vi "Lab Panel V5.26.vi"() -> ()   [LabVIEW 2017]
uses:
  <vilib>/platform/TimedLoop/XDataNode/XDataNode.xnode
  <vilib>/Platform/TimedLoop/XDataNode/nitl_modes.ctl
  <vilib>/Platform/TimedLoop/XDataNode/XDNodeRunTimeDep.lvlib
  <vilib>/Platform/TimedLoop/XDataNode/wakeup.ctl
  <vilib>/Platform/TimedLoop/XDataNode/timing_clust.ctl
  Global 1.vi
  Global display 1.vi
  Global display 3.vi
  Global display 2.vi
  Global display 4.vi
panel:
  out "Simulate IND":bool
  out "Amb Tp":dbl format="%#.0f"
  out "Tp Up":dbl
  out "network error":bool
  out "TEMP":bool
  out "AI":bool
  in  "stop all":bool
  in  "ADMIN":bool
  in  "Tab Control 2":T1(tab)
  out "SIG LAB05-2":T2 {"PF" format="%.2f"; "AMPS" format="%.1f"}
  out "SIG LAB05-1":T2 {"PF" format="%.2f"; "AMPS" format="%.1f"}
  out "SIG LAB04-2":T2 {"PF" format="%.2f"; "AMPS" format="%.1f"}
  out "SIG LAB04-1":T2 {"PF" format="%.2f"; "AMPS" format="%.1f"}
  out "SIG LAB03-2":T2 {"PF" format="%.2f"; "AMPS" format="%.1f"}
  out "SIG LAB03-1":T2 {"PF" format="%.2f"; "AMPS" format="%.1f"}
  out "SIG LAB02-2":T2 {"PF" format="%.2f"; "AMPS" format="%.1f"}
  in  "RUN LAB01-1":bool
  in  "O/I  LAB05-1":bool
  in  "O/I  LAB05-2":bool
  in  "O/I  LAB04-1":bool
  in  "O/I  LAB04-2":bool
  in  "O/I  LAB02-1":bool
  in  "O/I  LAB02-2":bool
  in  "O/I  LAB01-2":bool
  in  "O/I  LAB01-1":bool
  in  "O/I  LAB03-1":bool
  in  "RUN LAB05-2":bool
  in  "RUN LAB05-1":bool
  in  "RUN LAB04-2":bool
  in  "RUN LAB04-1":bool
  in  "RUN LAB03-2":bool
  in  "RUN LAB03-1":bool
  in  "RUN LAB02-2":bool
  in  "RUN LAB02-1":bool
  in  "RUN LAB01-2":bool
  in  "SELECT LAB05-2":T3(radio)
  in  "SELECT LAB05-1":T3(radio)
  in  "SELECT LAB04-2":T3(radio)
  in  "SELECT LAB04-1":T3(radio)
  in  "SELECT LAB03-2":T3(radio)
  in  "SELECT LAB03-1":T3(radio)
  in  "SELECT LAB02-2":T3(radio)
  in  "SELECT LAB02-1":T3(radio)
  in  "SELECT LAB01-2":T3(radio)
  in  "SELECT LAB01-1":T3(radio)
  in  "O/I  LAB03-2":bool
  out "SIG LAB01-1":T2 {"PF" format="%.2f"; "AMPS" format="%.1f"}
  out "SIG LAB01-2":T2 {"PF" format="%.2f"; "AMPS" format="%.1f"}
  out "SIG LAB02-1":T2 {"PF" format="%.2f"; "AMPS" format="%.1f"}
  out "DISP LAB05-2":T4 {"MINS" format="%.2g"}
  out "DISP LAB05-1":T4 {"MINS" format="%.2g"}
  out "DISP LAB04-2":T4 {"MINS" format="%.2g"}
  out "DISP LAB04-1":T4 {"MINS" format="%.2g"}
  out "DISP LAB03-2":T4 {"MINS" format="%.2g"}
  out "DISP LAB03-1":T4 {"MINS" format="%.2g"}
  in  "SET LAB05-2":T5={"NAME"="", "DESCRIPTION"="", "CYCLES"=5.0, "T-RISE mins"=0.0, "T-RISE deg C"=0.0} {"CYCLES" min=5.0 step=1.0}
  in  "SET LAB05-1":T5={"NAME"="", "DESCRIPTION"="", "CYCLES"=5.0, "T-RISE mins"=0.0, "T-RISE deg C"=0.0} {"CYCLES" min=5.0 step=1.0}
  in  "SET LAB04-2":T5={"NAME"="", "DESCRIPTION"="", "CYCLES"=5.0, "T-RISE mins"=0.0, "T-RISE deg C"=0.0} {"CYCLES" min=5.0 step=1.0}
  in  "SET LAB04-1":T5={"NAME"="", "DESCRIPTION"="", "CYCLES"=5.0, "T-RISE mins"=0.0, "T-RISE deg C"=0.0} {"CYCLES" min=5.0 step=1.0}
  in  "SET LAB03-2":T5={"NAME"="", "DESCRIPTION"="", "CYCLES"=5.0, "T-RISE mins"=0.0, "T-RISE deg C"=0.0} {"CYCLES" min=5.0 step=1.0}
  in  "SET LAB03-1":T5={"NAME"="", "DESCRIPTION"="", "CYCLES"=5.0, "T-RISE mins"=0.0, "T-RISE deg C"=0.0} {"CYCLES" min=5.0 step=1.0}
  out "DISP LAB02-2":T4 {"MINS" format="%.2g"}
  out "DISP LAB02-1":T4 {"MINS" format="%.2g"}
  in  "SET LAB02-2":T5={"NAME"="", "DESCRIPTION"="", "CYCLES"=5.0, "T-RISE mins"=0.0, "T-RISE deg C"=0.0} {"CYCLES" min=5.0 step=1.0}
  in  "SET LAB02-1":T5={"NAME"="", "DESCRIPTION"="", "CYCLES"=5.0, "T-RISE mins"=0.0, "T-RISE deg C"=0.0} {"CYCLES" min=5.0 step=1.0}
  out "RESULT LAB05-2":bool
  out "RESULT LAB05-1":bool
  out "RESULT LAB04-2":bool
  out "RESULT LAB04-1":bool
  out "RESULT LAB03-2":bool
  out "RESULT LAB03-1":bool
  out "RESULT LAB02-2":bool
  out "RESULT LAB02-1":bool
  out "RESULT LAB01-2":bool
  out "RESULT LAB01-1":bool
  in  "SET LAB01-1":T5={"NAME"="", "DESCRIPTION"="", "CYCLES"=5.0, "T-RISE mins"=0.0, "T-RISE deg C"=0.0} {"CYCLES" min=5.0 step=1.0}
  in  "SET LAB01-2":T5={"NAME"="", "DESCRIPTION"="", "CYCLES"=5.0, "T-RISE mins"=0.0, "T-RISE deg C"=0.0} {"CYCLES" min=5.0 step=1.0}
  out "DISP LAB01-1":T4 {"MINS" format="%.2g"}
  out "DISP LAB01-2":T4 {"MINS" format="%.2f"}
  out "TEMP RISE LAB05-2":cluster{"TL":dbl, "TN":dbl}
  out "TEMP RISE LAB05-1":cluster{"TL":dbl, "TN":dbl}
  out "TEMP RISE LAB04-2":cluster{"TL":dbl, "TN":dbl}
  out "TEMP RISE LAB04-1":cluster{"TL":dbl, "TN":dbl}
  out "TEMP RISE LAB03-2":cluster{"TL":dbl, "TN":dbl}
  out "TEMP RISE LAB03-1":cluster{"TL":dbl, "TN":dbl}
  out "TEMP RISE LAB02-2":cluster{"TL":dbl, "TN":dbl}
  out "TEMP RISE LAB02-1":cluster{"TL":dbl, "TN":dbl}
  out "TEMP RISE LAB01-2":cluster{"TL":dbl, "TN":dbl}
  out "TEMP RISE LAB01-1":cluster{"TL":dbl, "TN":dbl}
  out "JIG LAB05-2":bool
  out "JIG LAB05-1":bool
  out "JIG LAB04-2":bool
  out "JIG LAB04-1":bool
  out "JIG LAB03-2":bool
  out "JIG LAB03-1":bool
  out "JIG LAB02-2":bool
  out "JIG LAB02-1":bool
  out "JIG LAB01-2":bool
  out "JIG LAB01-1":bool
  out "TEMP START LAB01-1":cluster{"TL":dbl, "TN":dbl}
  out "TEMP START LAB02-1":cluster{"TL":dbl, "TN":dbl}
  out "TEMP START LAB03-1":cluster{"TL":dbl, "TN":dbl}
  out "TEMP START LAB04-1":cluster{"TL":dbl, "TN":dbl}
  out "TEMP START LAB01-2":cluster{"TL":dbl, "TN":dbl}
  out "TEMP START LAB02-2":cluster{"TL":dbl, "TN":dbl}
  out "TEMP START LAB03-2":cluster{"TL":dbl, "TN":dbl}
  out "TEMP START LAB04-2":cluster{"TL":dbl, "TN":dbl}
  out "TEMP START LAB05-2":cluster{"TL":dbl, "TN":dbl}
  out "TEMP START LAB05-1":cluster{"TL":dbl, "TN":dbl}
  out "LOG LAB05-2":string
  out "LOG LAB04-2":string
  out "LOG LAB03-2":string
  out "LOG LAB02-2":string
  out "LOG LAB01-2":string
  out "LOG LAB05-1":string
  out "LOG LAB04-1":string
  out "LOG LAB03-1":string
  out "LOG LAB02-1":string
  out "LOG LAB01-1":string
  in  "Tab charts":T6(tab)
  out "LAB01 VOLTS":dynamicdata(graph)
  out "LAB01 AMPS":dynamicdata(graph)
  out "LAB01 deg C":dynamicdata(graph)
  out "LAB02 VOLTS":dynamicdata(graph)
  out "LAB02 AMPS":dynamicdata(graph)
  out "LAB02 deg C":dynamicdata(graph)
  out "LAB03 VOLTS":dynamicdata(graph)
  out "LAB03 AMPS":dynamicdata(graph)
  out "LAB03 deg C":dynamicdata(graph)
  out "LAB04 VOLTS":dynamicdata(graph)
  out "LAB04 AMPS":dynamicdata(graph)
  out "LAB04 deg C":dynamicdata(graph)
  out "LAB05 VOLTS":dynamicdata(graph)
  out "LAB05 AMPS":dynamicdata(graph)
  out "LAB05 deg C":dynamicdata(graph)
  out "Reset Error":bool
  out "Error Temp":bool
  out "Er USB#2":dbl
  out "Er USB#1":dbl
  out "Er USB#0":dbl
  out "Resets Done":dbl
  out "Error USB #2":bool
  out "Error USB #1":bool
  out "Error USB #0":bool
  in  "MAIL SETTINGS":T7
  out "MAIL REPORT":string
  in  "TO (string):":string
  in  "Send Mail Now":bool
  in  "Auto Mail Send":bool
  in  "Network Directory":path
  in  "JIG ON TIME (S)":dbl=1.0 min=1.0 max=10.0 step=0.5 format="%.1g"
  in  "JIG OFF TIME (S)":dbl=2.0 min=2.0 max=10.0 step=0.5 format="%.1g"
  in  "Reset Measuring":bool
  in  "Read Temp":bool
  out "JIG RELAY CYCLES":T8
  out "ON L05-2":cluster{"amps":dbl, "volts":dbl, "pf":dbl}
  out "ON L05-1":cluster{"amps":dbl, "volts":dbl, "pf":dbl}
  out "FAIL LAB05-2":cluster{"LO":dbl, "HI":dbl}
  out "FAIL LAB05-1":cluster{"LO":dbl, "HI":dbl}
  out "FAIL LAB04-2":cluster{"LO":dbl, "HI":dbl}
  out "FAIL LAB04-1":cluster{"LO":dbl, "HI":dbl}
  out "FAIL LAB03-2":cluster{"LO":dbl, "HI":dbl}
  out "FAIL LAB03-1":cluster{"LO":dbl, "HI":dbl}
  out "FAIL LAB02-2":cluster{"LO":dbl, "HI":dbl}
  out "FAIL LAB02-1":cluster{"LO":dbl, "HI":dbl}
  out "FAIL LAB01-2":cluster{"LO":dbl, "HI":dbl}
  out "FAIL LAB01-1":cluster{"LO":dbl, "HI":dbl}
  out "ON L01-1":cluster{"amps":dbl, "volts":dbl, "pf":dbl}
  out "ON L01-2":cluster{"amps":dbl, "volts":dbl, "pf":dbl}
  out "ON L02-1":cluster{"amps":dbl, "volts":dbl, "pf":dbl}
  out "ON L02-2":cluster{"amps":dbl, "volts":dbl, "pf":dbl}
  out "ON L03-1":cluster{"amps":dbl, "volts":dbl, "pf":dbl}
  out "ON L03-2":cluster{"amps":dbl, "volts":dbl, "pf":dbl}
  out "ON L04-1":cluster{"amps":dbl, "volts":dbl, "pf":dbl}
  out "ON L04-2":cluster{"amps":dbl, "volts":dbl, "pf":dbl}
  out "TEMP LA05":T9
  out "TEMP LA04":T9
  out "TEMP LA03":T9
  out "TEMP LA02":T9
  out "TEMP LA01":T9
  out "Ref deg C":dbl format="%#.0f"
  out "Temp read loop":dbl
  out "AI Task":bool
  out "AI Task2":dbl
  out "AI Task1":dbl
  out "AI Task0":dbl
  out "Total USB resets":dbl
  in  "Auto Reset":bool
  in  "Mail Test File To:":string
  in  "Mail Test Fail":bool
  out "graph flag":bool
  in  "Temp Test Cal":dbl
  in  "Amps Fail level":dbl
  in  "Fail Loops":dbl
  out "Save JC":bool
  in  "Simulate":bool
  in  "Temp Value":dbl
  in  "Temp Delay Lps":dbl
  in  "SAMPLES":dbl
  in  "RATE (Hz)":dbl
  in  "JIG TEST":T10
  in  "C drive data root dir":path
  out "run lab05-2":bool
  out "run lab05-1":bool
  out "run lab04-2":bool
  out "run lab04-1":bool
  out "run lab03-2":bool
  out "run lab03-1":bool
  out "run lab02-2":bool
  out "run lab02-1":bool
  out "run lab01-2":bool
  out "run lab01-1":bool
  in  "Tab Control":T11(tab)
  out "LAB01-2 (GRAPH)":dynamicdata(graph)
  out "LAB01-1 (GRAPH)":dynamicdata(graph)
  out "LAB02-2 (GRAPH)":dynamicdata(graph)
  out "LAB02-1 (GRAPH)":dynamicdata(graph)
  out "LAB03-2 (GRAPH)":dynamicdata(graph)
  out "LAB03-1 (GRAPH)":dynamicdata(graph)
  out "LAB04-2 (GRAPH)":dynamicdata(graph)
  out "LAB04-1 (GRAPH)":dynamicdata(graph)
  out "LAB05-2 (GRAPH)":dynamicdata(graph)
  out "LAB05-1 (GRAPH)":dynamicdata(graph)
  out "Any Test Running":bool
  out "Read Time":dbl
  out "LAB05 TEMP":T12
  out "LAB04 TEMP":T12
  out "LAB02 TEMP":T12
  out "LAB01 TEMP":T12
  out "LAB03 TEMP":T12
  out "LAB05-TP":bool
  out "LAB04-TP":bool
  out "LAB03-TP":bool
  out "LAB02-TP":bool
  out "LAB01-TP":bool
  out "Analog error":bool
  out "USB OUT 0":bool[](array[boolean])
  out "USB OUT 1":bool[](array[boolean])
  out "USB OUT 2":bool[](array[boolean])
  in  "Ambient Volts":dbl format="%.2f"
  in  "PF":dbl min=0.0 max=1.0 step=0.1 format="%#.1f"
  in  "VOLTS":dbl
  in  "OFF amps":dbl min=0.0 max=100.0 step=0.1 format="%#.1f"
  in  "ON amps":dbl
  in  "LAB deg C":T13
  out "AI data 0":waveform(dbl)[](array[waveform])
  out "AI data 1":waveform(dbl)[](array[waveform])
  out "AI data 2":waveform(dbl)[](array[waveform])
  out "AI Error":errorcluster[](array[cluster])
  out "AI loop time":dbl format="%.6g"
  out "loops":dbl
  in  "SAMPLES 2":dbl
  out "on loops":dbl format="%#.0f"
  out "off loops":dbl format="%#.0f"
  out "jig cycle":dbl
  out "TDMS LAB01-1":refnum<k34>
  out "data file error":errorcluster
  out "TDMS LAB02-1":refnum<k34>
  out "TDMS LAB01-2":refnum<k34>
  out "TDMS LAB02-2":refnum<k34>
  out "TDMS LAB03-1":refnum<k34>
  out "TDMS LAB03-2":refnum<k34>
  out "TDMS LAB04-1":refnum<k34>
  out "TDMS LAB04-2":refnum<k34>
  out "TDMS LAB05-1":refnum<k34>
  out "TDMS LAB05-2":refnum<k34>
  out "mail control":string
  out "File Time Stamp":timestamp
  in  "stop":bool
  in  "Select COM port":refnum<visa-resource-name>="COM6"
  out "COM port":refnum<visa-resource-name>="COM6"
  out "deg C (volts)":dbl
  out "TEMP REF cal":dbl
  out "CAL LAB01":T14 {"2 (TN) cal" min=0.0 step=0.01 format="%.2f"; "2 (TL) cal" min=0.0 step=0.01 format="%.2f"; "2 (PF) cal" min=0.0 step=0.01 format="%.2f"; "2 (V) cal" min=0.0 step=0.01 format="%.2f"; "2 (A) cal" min=0.0 step=0.01 format="%.2f"; "1 (TN) cal" min=0.0 step=0.01 format="%.2f"; "1 (TL) cal" min=0.0 step=0.01 format="%.2f"; "1 (PF) cal" min=0.0 step=0.01 format="%.2f"; "1 (V) cal" min=0.0 step=0.01 format="%.2f"; "1  (A) cal" min=0.0 step=0.01 format="%.2f"}
  out "CAL LAB03":T14 {"2 (TN) cal" min=0.0 step=0.01 format="%.2f"; "2 (TL) cal" min=0.0 step=0.01 format="%.2f"; "2 (PF) cal" min=0.0 step=0.01 format="%.2f"; "2 (V) cal" min=0.0 step=0.01 format="%.2f"; "2 (A) cal" min=0.0 step=0.01 format="%.2f"; "1 (TN) cal" min=0.0 step=0.01 format="%.2f"; "1 (TL) cal" min=0.0 step=0.01 format="%.2f"; "1 (PF) cal" min=0.0 step=0.01 format="%.2f"; "1 (V) cal" min=0.0 step=0.01 format="%.2f"; "1  (A) cal" min=0.0 step=0.01 format="%.2f"}
  out "CAL LAB02":T15 {"2 (TN) cal" min=0.0 step=0.01 format="%.2f"; "2 (TL) cal" min=0.0 step=0.01 format="%.2f"; "2 (PF) cal" min=0.0 step=0.01 format="%.2f"; "2 (V) cal" min=0.0 step=0.01 format="%.2f"; "2 (A) cal" min=0.0 step=0.01 format="%.2f"; "1 (TN) cal" min=0.0 step=0.01 format="%.2f"; "1 (TL) cal" min=0.0 step=0.01 format="%.2f"; "1 (PF) cal" min=0.0 step=0.01 format="%.2f"; "1 (V) cal" min=0.0 step=0.01 format="%.2f"; "1 (A) cal" min=0.0 step=0.01 format="%.2f"}
  out "CAL LAB05":T14 {"2 (TN) cal" min=0.0 step=0.01 format="%.2f"; "2 (TL) cal" min=0.0 step=0.01 format="%.2f"; "2 (PF) cal" min=0.0 step=0.01 format="%.2f"; "2 (V) cal" min=0.0 step=0.01 format="%.2f"; "2 (A) cal" min=0.0 step=0.01 format="%.2f"; "1 (TN) cal" min=0.0 step=0.01 format="%.2f"; "1 (TL) cal" min=0.0 step=0.01 format="%.2f"; "1 (PF) cal" min=0.0 step=0.01 format="%.2f"; "1 (V) cal" min=0.0 step=0.01 format="%.2f"; "1  (A) cal" min=0.0 step=0.01 format="%.2f"}
  out "CAL LAB04":T14 {"2 (TN) cal" min=0.0 step=0.01 format="%.2f"; "2 (TL) cal" min=0.0 step=0.01 format="%.2f"; "2 (PF) cal" min=0.0 step=0.01 format="%.2f"; "2 (V) cal" min=0.0 step=0.01 format="%.2f"; "2 (A) cal" min=0.0 step=0.01 format="%.2f"; "1 (TN) cal" min=0.0 step=0.01 format="%.2f"; "1 (TL) cal" min=0.0 step=0.01 format="%.2f"; "1 (PF) cal" min=0.0 step=0.01 format="%.2f"; "1 (V) cal" min=0.0 step=0.01 format="%.2f"; "1  (A) cal" min=0.0 step=0.01 format="%.2f"}
  out "cal file error out":errorcluster
  in  "SET (cal)":bool
  out "AI Data 0":waveform(dbl)[](graph)
  out "AI Data 1":waveform(dbl)[](graph)
  out "AI Data 2":waveform(dbl)[](graph)
  # "LAB01"
  # "LAB02"
  # "LAB03"
  # "LAB04"
  # "LAB05"
  # "LAB01"
  # "LAB02"
  # "LAB03"
  # "LAB04"
  # "LAB05"
  # "PANEL ID / DATE / TIME / NAME / DESCRIPTION / CYCLES / TEST TIME / STATUS"
  # "PANEL ID / DATE / TIME / NAME / DESCRIPTION / CYCLES / TEST TIME / STATUS"
  # "(Enter recipients address seperated by comma)"
  # "JIG SET"
  # "Temperature circuits \ndetected at start up."
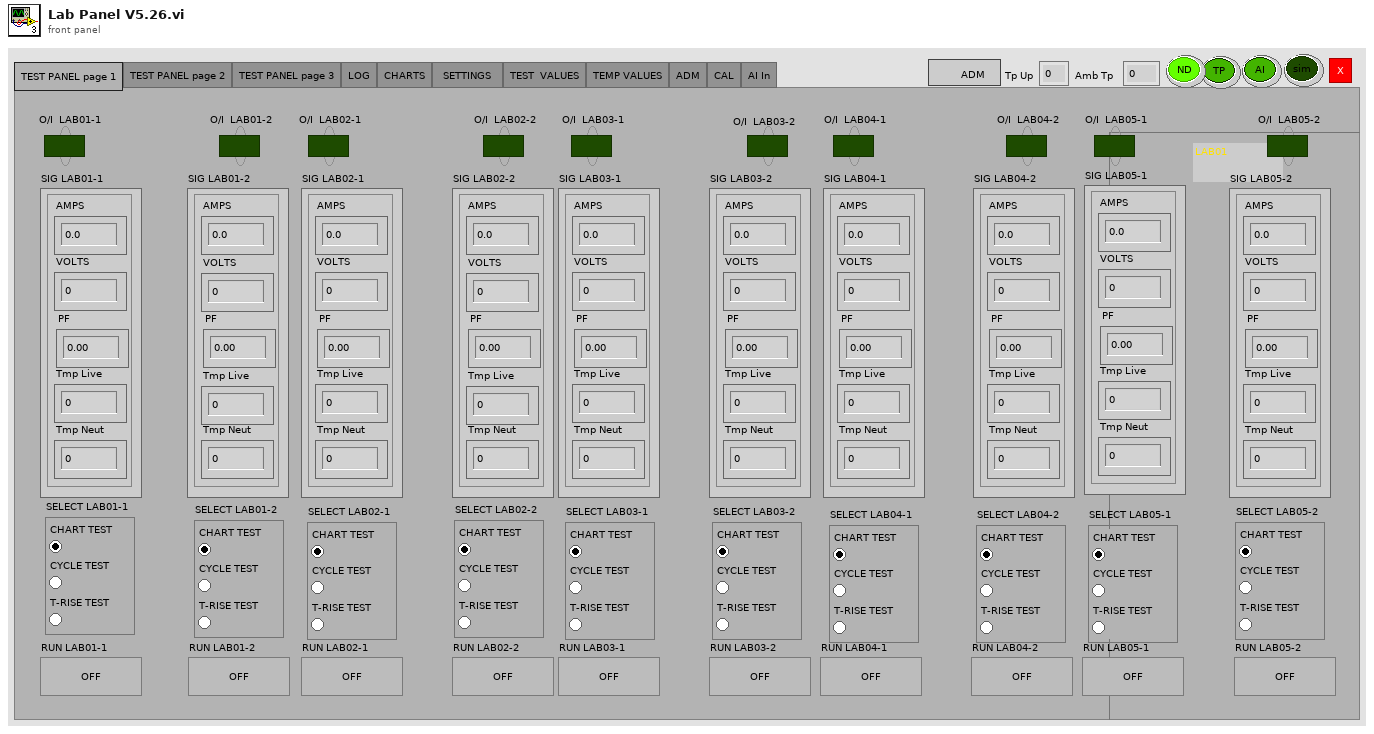
[diagram p1: front panel]
types:
  T1 = enum32{"TEST PANEL page 1", "TEST PANEL page 2", "TEST PANEL page 3", "LOG", "CHARTS", "SETTINGS   ", "TEST  VALUES", "TEMP VALUES", "ADM", "CAL", "AI In"}
  T2 = cluster{"AMPS":dbl, "VOLTS":dbl, "PF":dbl, "Tmp Live":dbl, "Tmp Neut":dbl}
  T3 = enum32{"CHART TEST", "CYCLE TEST", "T-RISE TEST"}
  T4 = cluster{"CYCLE":dbl, "MINS":dbl, "STATUS":string}
  T5 = cluster{"NAME":string, "DESCRIPTION":string, "CYCLES":dbl, "T-RISE mins":dbl, "T-RISE deg C":dbl}
  T6 = enum32{"LAB01", "LAB02", "LAB03", "LAB04", "LAB05"}
  T7 = cluster{"OUT SERVER ADDRESS":string, "FROM ACCOUNT":string, "USER NAME":string, "PASSWORD":string, "TEST MAIL":bool, "TEST MAIL STATUS":string, "mail error":errorcluster}
  T8 = cluster{"LAB01-1":dbl, "LAB01-2":dbl, "LAB02-1":dbl, "LAB02-2":dbl, "LAB03-1":dbl, "LAB03-2":dbl, "LAB04-1":dbl, "LAB04-2":dbl, "LAB05-1":dbl, "LAB05-2":dbl}
  T9 = cluster{"TL-1":dbl, "TN-1":dbl, "TL-2":dbl, "TN-2":dbl, "TL -1COUNT":dbl, "TN-1 COUNT":dbl, "TL-2 COUNT":dbl, "TN-2 COUNT":dbl}
  T10 = cluster{" LAB01-1":bool, " LAB01-2":bool, "LAB02-1":bool, " LAB02-2":bool, "LAB03-1":bool, "LAB03-2":bool, "LAB04-1":bool, "LAB04-2":bool, "LAB05-1":bool, "LAB05-2":bool}
  T11 = enum32{"LAB01", "LAB02", "LAB03", "LAB04", "LAB05", "TEMPERATURE", "GENERAL INFO", "Simulate", "AI Data Out"}
  T12 = cluster{"T1 Live":dbl, "T1 Neut":dbl, "T2 Live":dbl, "T2 Neut":dbl, "ID":dbl, "ER":dbl}
  T13 = cluster{"1 TL":dbl, "1 TN":dbl, "2 TL":dbl, "2 TN":dbl, "ID":dbl, "ER":dbl}
  T14 = cluster{"1  (A) cal":dbl, "1 (V) cal":dbl, "1 (PF) cal":dbl, "1 (TL) cal":dbl, "1 (TN) cal":dbl, "2 (A) cal":dbl, "2 (V) cal":dbl, "2 (PF) cal":dbl, "2 (TL) cal":dbl, "2 (TN) cal":dbl}
  T15 = cluster{"1 (A) cal":dbl, "1 (V) cal":dbl, "1 (PF) cal":dbl, "1 (TL) cal":dbl, "1 (TN) cal":dbl, "2 (A) cal":dbl, "2 (V) cal":dbl, "2 (PF) cal":dbl, "2 (TL) cal":dbl, "2 (TN) cal":dbl}
  T16 = enum8{"Enabled", "Disabled", "Disabled and Grayed Out"}
  T17 = enum16{"open", "replace", "create", "open or create", "replace or create", "replace or create with confirmation"}
  T18 = typedef "XDNodeRunTimeDep.lvlib/timing_clust.ctl" = cluster{"Expected End [f-1]":u64, "Actual End [f-1]":u64, "Finished Late? [f-1]":bool, "Expected End [i-1]":u64, "Actual End [i-1]":u64, "Finished Late? [i-1]":bool, "Expected Start [i]":u64, "Actual Start [i]":u64, "Expected Start [f]":u64, "Actual Start [f]":u64, "Source Name":string, "Structure Name":string, "Period":i64, "Deadline":i64, "Offset":i64, "Start":i64, "Priority":i32, "Timeout":i32, "Mode":T19, "Wakeup Reason":T20, "Error":errorcluster, "Source Type":string, "Secondary Source Type":string, "Global End Time":u64, "Global Start Time":u64, "Frame Duration":u64, "Iteration Duration":u64, "Assigned CPU":i32, "I/O Scan Engine Mode":u32}
  T19 = typedef "XDNodeRunTimeDep.lvlib/nitl_modes.ctl" = enum32{"No Change", "Process missed periods, maintain original phase", "Discard missed periods, maintain original phase", "Process missed periods, ignore original phase", "Discard missed periods, ignore original phase"}
  T20 = typedef "XDNodeRunTimeDep.lvlib/wakeup.ctl" = enum32{"Normal", "Aborted", "Asynchronous wakeup", "Timing source error", "Timed loop error", "Timeout"}
  T21 = enum16{"open", "open or create", "create or replace", "create", "open (read-only)"}
  T22 = cluster{"SET LAB01-1":cluster{"NAME":string, "DESCRIPTION":string, "CYCLES":dbl, "T-RISE mins":dbl, "T-RISE deg C":dbl}, "SET LAB01-2":cluster{"NAME":string, "DESCRIPTION":string, "CYCLES":dbl, "T-RISE mins":dbl, "T-RISE deg C":dbl}, "SET LAB02-1":cluster{"NAME":string, "DESCRIPTION":string, "CYCLES":dbl, "T-RISE mins":dbl, "T-RISE deg C":dbl}, "SET LAB02-2":cluster{"NAME":string, "DESCRIPTION":string, "CYCLES":dbl, "T-RISE mins":dbl, "T-RISE deg C":dbl}, "SET LAB03-1":cluster{"NAME":string, "DESCRIPTION":string, "CYCLES":dbl, "T-RISE mins":dbl, "T-RISE deg C":dbl}, "SET LAB03-2":cluster{"NAME":string, "DESCRIPTION":string, "CYCLES":dbl, "T-RISE mins":dbl, "T-RISE deg C":dbl}, "SET LAB04-1":cluster{"NAME":string, "DESCRIPTION":string, "CYCLES":dbl, "T-RISE mins":dbl, "T-RISE deg C":dbl}, "SET LAB04-2":cluster{"NAME":string, "DESCRIPTION":string, "CYCLES":dbl, "T-RISE mins":dbl, "T-RISE deg C":dbl}, "SET LAB05-1":cluster{"NAME":string, "DESCRIPTION":string, "CYCLES":dbl, "T-RISE mins":dbl, "T-RISE deg C":dbl}, "SET LAB05-2":cluster{"NAME":string, "DESCRIPTION":string, "CYCLES":dbl, "T-RISE mins":dbl, "T-RISE deg C":dbl}, "Network Directory":path, "C drive data root dir":path, "RATE (Hz)":dbl, "SAMPLES":dbl, "Select COM port":refnum<visa-resource-name>, "Temp Delay Lps":dbl, "Temp Value":dbl, "Fail Loops":dbl, "Temp Test Cal":dbl, "Amps Fail level":dbl, "Mail Test File To:":string, "Mail Test Fail":bool, "SAMPLES 2":dbl}
  T23 = cluster{"MAIL SETTINGS":cluster{"OUT SERVER ADDRESS":string, "FROM ACCOUNT":string, "USER NAME":string, "PASSWORD":string, "TEST MAIL":bool, "TEST MAIL STATUS":string, "mail error":errorcluster}, "Auto Mail Send":bool, string}
  T24 = cluster{"id1":bool, "id2":bool, "id3":bool, "id4":bool, "id5":bool}
  T25 = cluster{"T1":dbl, "T2":dbl, "T3":dbl, "T4":dbl, "ID":dbl, "ER":dbl}
  T26 = cluster{"STATUS":string, "OUT SERVER ADDRESS":string, "FROM ACCOUNT":string, "Mail Test File To:":string, "Mail Test Fail":bool}
  T27 = cluster{"LAB01-1 (A)":dbl, "LAB01-1 (V)":dbl, "LAB01-1 (PF)":dbl, "LAB01-2 (A)":dbl, "LAB01-2 (V)":dbl, "LAB01-2 (PF)":dbl}
  T28 = cluster{"LAB02-1 (A)":dbl, "LAB02-1 (V)":dbl, "LAB02-1 (PF)":dbl, "LAB02-2 (A)":dbl, "LAB02-2 (V)":dbl, "LAB02-2 (PF)":dbl}
  T29 = cluster{"LAB03-1 (A)":dbl, "LAB03-1 (V)":dbl, "LAB03-1 (PF)":dbl, "LAB03-2 (A)":dbl, "LAB03-2 (V)":dbl, "LAB03-2 (PF)":dbl}
  T30 = cluster{"LAB04-1 (A)":dbl, "LAB04-1 (V)":dbl, "LAB04-1 (PF)":dbl, "LAB04-2 (A)":dbl, "LAB04-2 (V)":dbl, "LAB04-2 (PF)":dbl}
  T31 = cluster{"LAB05-1 (A)":dbl, "LAB05-1 (V)":dbl, "LAB05-1 (PF)":dbl, "LAB05-2 (A)":dbl, "LAB05-2 (V)":dbl, "LAB05-2 (PF)":dbl}
  T32 = cluster{"OFF amps":dbl, "VOLTS":dbl, "PF":dbl, "OFF amps":dbl, "VOLTS":dbl, "PF":dbl}
  T33 = cluster{"FAIL LAB01-1":cluster{"LO":dbl, "HI":dbl}, "SIG LAB01-1":cluster{"AMPS":dbl, "VOLTS":dbl, "PF":dbl, "Tmp Live":dbl, "Tmp Neut":dbl}, "TEMP START LAB01-1":cluster{"TL":dbl, "TN":dbl}, "DISP LAB01-1":cluster{"CYCLE":dbl, "MINS":dbl, "STATUS":string}, "SET LAB01-1":cluster{"NAME":string, "DESCRIPTION":string, "CYCLES":dbl, "T-RISE mins":dbl, "T-RISE deg C":dbl}, "TDMS LAB01-1":refnum<k34>}
  T34 = cluster{"FAIL LAB01-2":cluster{"LO":dbl, "HI":dbl}, "SIG LAB01-2":cluster{"AMPS":dbl, "VOLTS":dbl, "PF":dbl, "Tmp Live":dbl, "Tmp Neut":dbl}, "TEMP START LAB01-2":cluster{"TL":dbl, "TN":dbl}, "DISP LAB01-2":cluster{"CYCLE":dbl, "MINS":dbl, "STATUS":string}, "SET LAB01-2":cluster{"NAME":string, "DESCRIPTION":string, "CYCLES":dbl, "T-RISE mins":dbl, "T-RISE deg C":dbl}, "TDMS LAB01-2":refnum<k34>}
  T35 = cluster{"FAIL LAB02-1":cluster{"LO":dbl, "HI":dbl}, "SIG LAB02-1":cluster{"AMPS":dbl, "VOLTS":dbl, "PF":dbl, "Tmp Live":dbl, "Tmp Neut":dbl}, "TEMP START LAB02-1":cluster{"TL":dbl, "TN":dbl}, "DISP LAB02-1":cluster{"CYCLE":dbl, "MINS":dbl, "STATUS":string}, "SET LAB02-1":cluster{"NAME":string, "DESCRIPTION":string, "CYCLES":dbl, "T-RISE mins":dbl, "T-RISE deg C":dbl}, "TDMS LAB02-1":refnum<k34>}
  T36 = cluster{"FAIL LAB02-2":cluster{"LO":dbl, "HI":dbl}, "SIG LAB02-2":cluster{"AMPS":dbl, "VOLTS":dbl, "PF":dbl, "Tmp Live":dbl, "Tmp Neut":dbl}, "TEMP START LAB02-2":cluster{"TL":dbl, "TN":dbl}, "DISP LAB02-2":cluster{"CYCLE":dbl, "MINS":dbl, "STATUS":string}, "SET LAB02-2":cluster{"NAME":string, "DESCRIPTION":string, "CYCLES":dbl, "T-RISE mins":dbl, "T-RISE deg C":dbl}, "TDMS LAB02-2":refnum<k34>}
  T37 = cluster{"FAIL LAB03-1":cluster{"LO":dbl, "HI":dbl}, "SIG LAB03-1":cluster{"AMPS":dbl, "VOLTS":dbl, "PF":dbl, "Tmp Live":dbl, "Tmp Neut":dbl}, "TEMP START LAB03-1":cluster{"TL":dbl, "TN":dbl}, "DISP LAB03-1":cluster{"CYCLE":dbl, "MINS":dbl, "STATUS":string}, "SET LAB03-1":cluster{"NAME":string, "DESCRIPTION":string, "CYCLES":dbl, "T-RISE mins":dbl, "T-RISE deg C":dbl}, "TDMS LAB03-1":refnum<k34>}
  T38 = cluster{"FAIL LAB03-2":cluster{"LO":dbl, "HI":dbl}, "SIG LAB03-2":cluster{"AMPS":dbl, "VOLTS":dbl, "PF":dbl, "Tmp Live":dbl, "Tmp Neut":dbl}, "TEMP START LAB03-2":cluster{"TL":dbl, "TN":dbl}, "DISP LAB03-2":cluster{"CYCLE":dbl, "MINS":dbl, "STATUS":string}, "SET LAB03-2":cluster{"NAME":string, "DESCRIPTION":string, "CYCLES":dbl, "T-RISE mins":dbl, "T-RISE deg C":dbl}, "TDMS LAB03-2":refnum<k34>}
  T39 = cluster{"FAIL LAB04-1":cluster{"LO":dbl, "HI":dbl}, "SIG LAB04-1":cluster{"AMPS":dbl, "VOLTS":dbl, "PF":dbl, "Tmp Live":dbl, "Tmp Neut":dbl}, "TEMP START LAB04-1":cluster{"TL":dbl, "TN":dbl}, "DISP LAB04-1":cluster{"CYCLE":dbl, "MINS":dbl, "STATUS":string}, "SET LAB04-1":cluster{"NAME":string, "DESCRIPTION":string, "CYCLES":dbl, "T-RISE mins":dbl, "T-RISE deg C":dbl}, "TDMS LAB04-1":refnum<k34>}
  T40 = cluster{"FAIL LAB04-2":cluster{"LO":dbl, "HI":dbl}, "SIG LAB04-2":cluster{"AMPS":dbl, "VOLTS":dbl, "PF":dbl, "Tmp Live":dbl, "Tmp Neut":dbl}, "TEMP START LAB04-2":cluster{"TL":dbl, "TN":dbl}, "DISP LAB04-2":cluster{"CYCLE":dbl, "MINS":dbl, "STATUS":string}, "SET LAB04-2":cluster{"NAME":string, "DESCRIPTION":string, "CYCLES":dbl, "T-RISE mins":dbl, "T-RISE deg C":dbl}, "TDMS LAB04-2":refnum<k34>}
  T41 = cluster{"FAIL LAB05-1":cluster{"LO":dbl, "HI":dbl}, "SIG LAB05-1":cluster{"AMPS":dbl, "VOLTS":dbl, "PF":dbl, "Tmp Live":dbl, "Tmp Neut":dbl}, "TEMP START LAB05-1":cluster{"TL":dbl, "TN":dbl}, "DISP LAB05-1":cluster{"CYCLE":dbl, "MINS":dbl, "STATUS":string}, "SET LAB05-1":cluster{"NAME":string, "DESCRIPTION":string, "CYCLES":dbl, "T-RISE mins":dbl, "T-RISE deg C":dbl}, "TDMS LAB05-1":refnum<k34>}
  T42 = cluster{"FAIL LAB05-2":cluster{"LO":dbl, "HI":dbl}, "SIG LAB05-2":cluster{"AMPS":dbl, "VOLTS":dbl, "PF":dbl, "Tmp Live":dbl, "Tmp Neut":dbl}, "TEMP START LAB05-2":cluster{"TL":dbl, "TN":dbl}, "DISP LAB05-2":cluster{"CYCLE":dbl, "MINS":dbl, "STATUS":string}, "SET LAB05-2":cluster{"NAME":string, "DESCRIPTION":string, "CYCLES":dbl, "T-RISE mins":dbl, "T-RISE deg C":dbl}, "TDMS LAB05-2":refnum<k34>}
  T43 = cluster{"MAIL SETTINGS":cluster{"OUT SERVER ADDRESS":string, "FROM ACCOUNT":string, "USER NAME":string, "PASSWORD":string, "TEST MAIL":bool, "TEST MAIL STATUS":string, "mail error":errorcluster}, "Auto Mail Send":bool, "TO (string):":string}
  T44 = cluster{"TP1-L":dbl, "TP1-N":dbl, "TP2-L":dbl, "TP2-N":dbl, "TP1-L COUNT":dbl, "TP1-N COUNT":dbl, "TP2-L COUNT":dbl, "TP2-N COUNT":dbl}
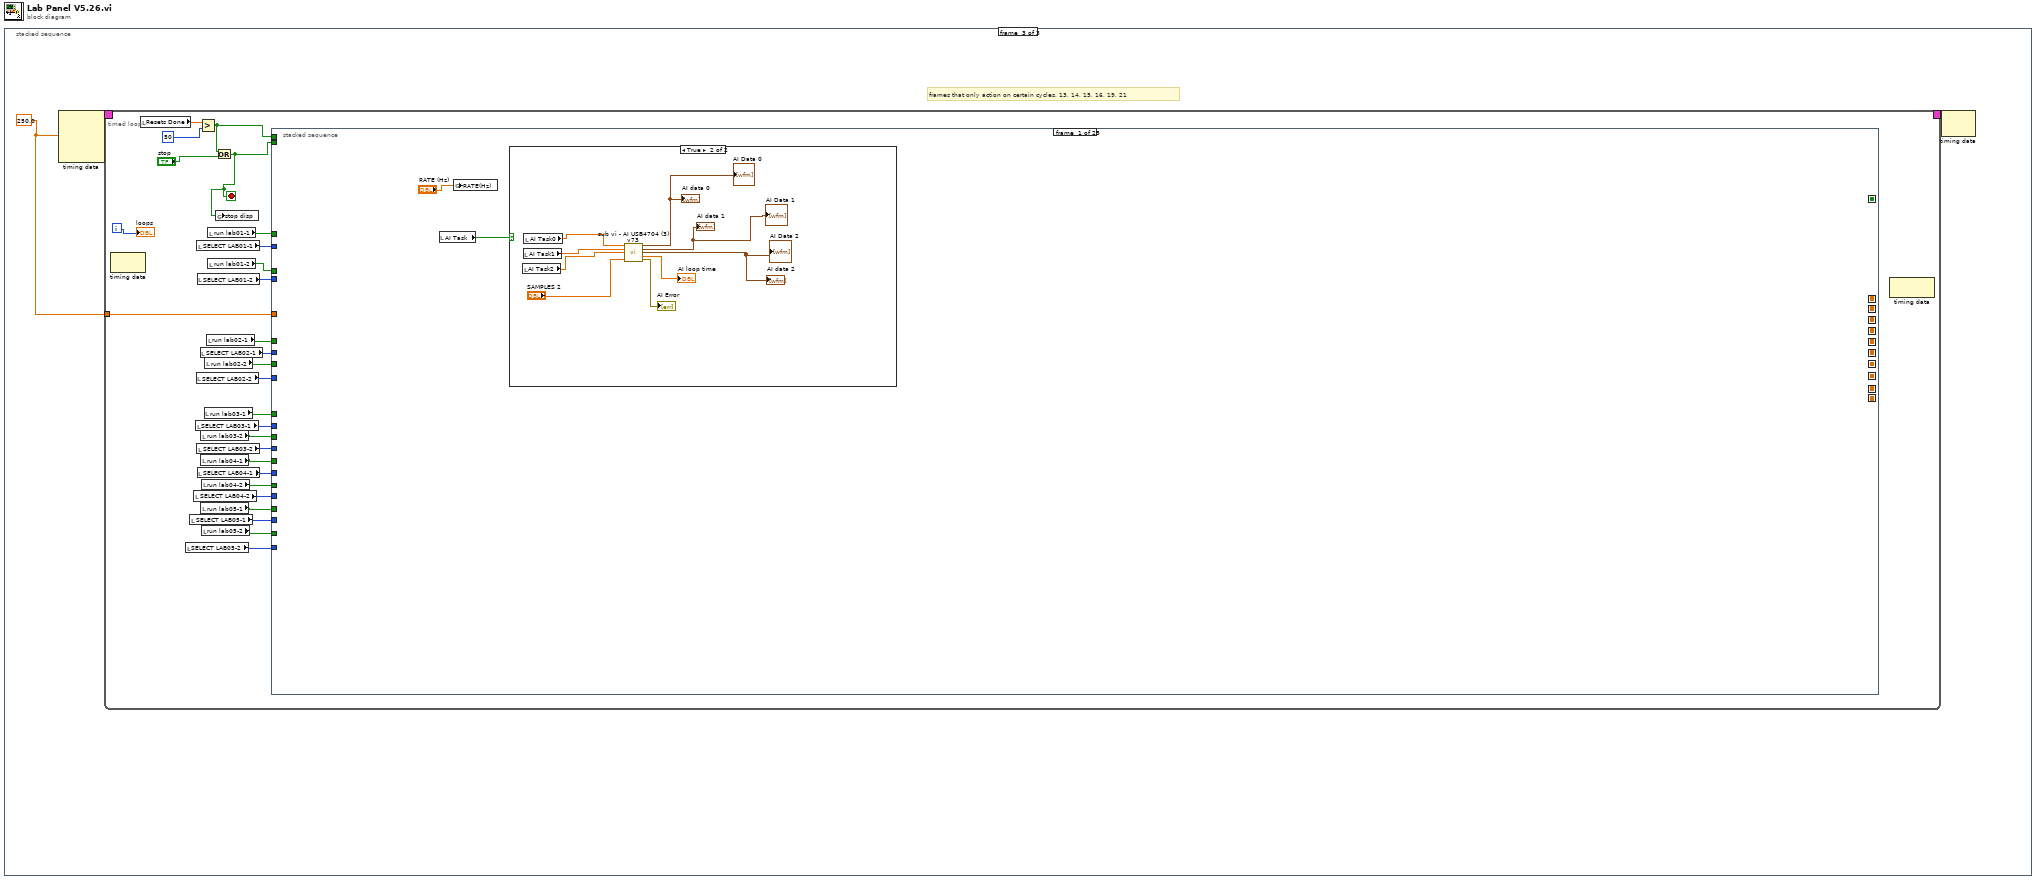
[diagram p0: block diagram]
diagram:
  n1 = stacked-sequence {
    frame #0 {
      n2 = local write "Save JC"(FALSE) -> ()
      "jig cycle" <- 0
    }
    frame #1 {
      # "do 1st time set up"
      n3 = stacked-sequence {
        frame #0 {
          # "check for simulate mode"
          n4 = call "subvi-simulate v1.vi"() -> ("Sim"=w3:bool)  [unwired: 11 in]
          n5 = case shown="True" w3 {
            frame False {
            }
            frame True {
              n6 = local write "Simulate"(TRUE) -> ()
            }
          }
        }
        frame #1 {
          n7 = local read "Simulate"() -> (w5:bool)
          n8 = case shown="False" w5 {
            frame False {
              # "RESET USB AND TEMPERATURE CIRCUITS"
              n9 = call "Reset USB&temp v 1.vi"() -> ()  [unwired: 11 in, 1 out]
            }
            frame True {
            }
          }
        }
        frame #2 {
          # "disable front panel while 1st time set up is being done"
          n10 = disable-structure shown="Enabled" {
            frame Enabled {
              n11 = property on="Tab Control 2" class="TabCtl (strict)"() -> ("Pages"=w12:refnum<vi>[])  [unwired: 2 in, 2 out]
              n12 = Index Array(array=w12, index=8) -> (element=w10:refnum<vi>)
              n13 = property class="Page"(reference=w10, "PageVis"=FALSE) -> ()  [unwired: 1 in, 2 out]
            }
            frame Disabled {
            }
          }
          n14 = property on="Tab Control 2" class="TabCtl (strict)"("Value"=0) -> ()  [unwired: 2 in, 2 out]
          n15 = local write "ADMIN"(FALSE) -> ()
          n16 = property on="Tab Control 2" class="TabCtl (strict)"("DisabledEnum"=T16."Disabled and Grayed Out" ("Disabled")) -> ()  [unwired: 2 in, 2 out]
        }
        frame #3 {
          # "get calibration values"
          n17 = call "sub vi - get calibration values v1.vi"() -> ("TEMP REF CAL"=w13:dbl, "LAB01 (CAL)"=→"CAL LAB01":T14, "LAB02 (CAL)"=→"CAL LAB02":T15, "LAB03 (CAL)"=→"CAL LAB03":T14, "LAB04 (CAL)"=→"CAL LAB04":T14, "calibration file error out"=→"cal file error out":errorcluster, "LAB05 (CAL)"=→"CAL LAB05":T14)  [unwired: 9 in]
          n18 = local write "TEMP REF cal"(w13) -> ()
        }
        frame #4 {
          # "get last saved test settings from file"
          n19 = local read "Network Directory"() -> (w44:path)
          n20 = local read "C drive data root dir"() -> (w42:path)
          n21 = local read "SET LAB05-2"() -> (w74:T5)
          n22 = local read "SAMPLES"() -> (w40:dbl)
          n23 = local read "SET LAB05-1"() -> (w75:T5)
          n24 = local read "RATE (Hz)"() -> (w41:dbl)
          n25 = local read "SET LAB04-2"() -> (w76:T5)
          n26 = local read "SET LAB03-2"() -> (w73:T5)
          n27 = local read "SET LAB04-1"() -> (w77:T5)
          n28 = local read "SET LAB03-1"() -> (w72:T5)
          n29 = local read "SET LAB02-2"() -> (w71:T5)
          n30 = local read "SET LAB02-1"() -> (w70:T5)
          n31 = local read "SET LAB01-2"() -> (w69:T5)
          n32 = local read "SET LAB01-1"() -> (w68:T5)
          n33 = local read "Select COM port"() -> (w37:refnum<visa-resource-name>)
          n34 = local read "Temp Delay Lps"() -> (w36:dbl)
          n35 = local read "Mail Test File To:"() -> (w26:string)
          n36 = local read "Temp Value"() -> (w35:dbl)
          n37 = local read "Temp Test Cal"() -> (w30:dbl)
          n38 = local read "Amps Fail level"() -> (w29:dbl)
          n39 = local read "Fail Loops"() -> (w32:dbl)
          n40 = local read "Mail Test Fail"() -> (w24:bool)
          n41 = local read "SAMPLES 2"() -> (w21:dbl)
          n42 = Bundle("SET LAB01-1"=w68, "SET LAB01-2"=w69, "SET LAB02-1"=w70, "SET LAB02-2"=w71, "SET LAB03-1"=w72, "SET LAB03-2"=w73, "SET LAB04-1"=w77, "SET LAB04-2"=w76, "SET LAB05-1"=w75, "SET LAB05-2"=w74, "Network Directory"=w44, "C drive data root dir"=w42, "RATE (Hz)"=w41, "SAMPLES"=w40, "Select COM port"=w37, "Temp Delay Lps"=w36, "Temp Value"=w35, "Fail Loops"=w32, "Temp Test Cal"=w30, "Amps Fail level"=w29, "Mail Test File To:"=w26, "Mail Test Fail"=w24, "SAMPLES 2"=w21) -> (w61:T22)  [unwired: 1 in]
          n43 = String To Path(string="c:\\crabtree\\Set Up\\") -> (path=w65:path)
          n44 = Build Path(base path=w65, name or relative path="settings.bin") -> (appended path=w63:path)
          n45 = Create Folder(path (use dialog)=w65) -> (error out=w67:errorcluster)  [unwired: 2 in, 2 out]
          n46 = call <vilib>:"Clear Errors.vi"("error in (no error)"=w67) -> ()  [unwired: 5 in, 2 out]
          n47 = Open/Create/Replace File(file path (use dialog)=w63) -> (refnum out=w60:refnum<file>, error out=w62:errorcluster)  [unwired: 5 in, 1 out]
          n48 = Read from Binary File(5:w61, 8:w62, 11:w60) -> (0:w57:errorcluster, 2:w59:T22, 3:w58:refnum<file>)  [unwired: 3 in, 1 out]
          n49 = Unbundle(w59) -> ("SET LAB01-1"=w55:T5, "SET LAB01-2"=w54:T5, "SET LAB02-1"=w53:T5, "SET LAB02-2"=w52:T5, "SET LAB03-1"=w51:T5, "SET LAB03-2"=w50:T5, "SET LAB04-1"=w49:T5, "SET LAB04-2"=w48:T5, "SET LAB05-1"=w47:T5, "SET LAB05-2"=w46:T5, "Network Directory"=w45:path, "C drive data root dir"=w43:path, "RATE (Hz)"=w38:dbl, "SAMPLES"=w39:dbl, "Select COM port"=w22:refnum<visa-resource-name>, "Temp Delay Lps"=w34:dbl, "Temp Value"=w33:dbl, "Fail Loops"=w31:dbl, "Temp Test Cal"=w28:dbl, "Amps Fail level"=w27:dbl, "Mail Test File To:"=w25:string, "Mail Test Fail"=w23:bool, "SAMPLES 2"=w20:dbl)
          n50 = Close File(refnum=w58, error in=w57) -> (error out=w56:errorcluster)  [unwired: 1 out]
          n51 = local write "data file error"(w56) -> ()
          n52 = local write "SAMPLES 2"(w20) -> ()
          n53 = local write "Temp Test Cal"(w28) -> ()
          n54 = local write "Amps Fail level"(w27) -> ()
          n55 = local write "Mail Test File To:"(w25) -> ()
          n56 = local write "Mail Test Fail"(w23) -> ()
          n57 = local write "Fail Loops"(w31) -> ()
          n58 = local write "Temp Delay Lps"(w34) -> ()
          n59 = local write "C drive data root dir"(w43) -> ()
          n60 = local write "Temp Value"(w33) -> ()
          n61 = local write "Network Directory"(w45) -> ()
          n62 = local write "SAMPLES"(w39) -> ()
          n63 = local write "RATE (Hz)"(w38) -> ()
          n64 = local write "SET LAB04-2"(w48) -> ()
          n65 = local write "SET LAB05-1"(w47) -> ()
          n66 = local write "SET LAB04-1"(w49) -> ()
          n67 = local write "SET LAB05-2"(w46) -> ()
          n68 = local write "SET LAB02-1"(w53) -> ()
          n69 = local write "SET LAB02-2"(w52) -> ()
          n70 = local write "SET LAB03-1"(w51) -> ()
          n71 = local write "SET LAB03-2"(w50) -> ()
          n72 = local write "SET LAB01-1"(w55) -> ()
          n73 = local write "SET LAB01-2"(w54) -> ()
          n74 = local write "Select COM port"(w22) -> ()
          n75 = global write "Global 1.vi" "COM port"(w22) -> ()
        }
        frame #5 {
          # "get total resets value from file"
          n76 = String To Path(string="c:\\crabtree\\Set Up\\") -> (path=w88:path)
          n77 = Build Path(base path=w88, name or relative path="USB resets.bin") -> (appended path=w81:path)
          n78 = Create Folder(path (use dialog)=w88) -> (error out=w80:errorcluster)  [unwired: 2 in, 2 out]
          n79 = call <vilib>:"Clear Errors.vi"("error in (no error)"=w80) -> ()  [unwired: 5 in, 2 out]
          n80 = Open/Create/Replace File(file path (use dialog)=w81, operation (0:open)=T17."open or create") -> (refnum out=w86:refnum<file>, error out=w85:errorcluster)  [unwired: 4 in, 1 out]
          n81 = local read "Total USB resets"() -> (w79:dbl)
          n82 = Read from Binary File(5:w79, 8:w85, 11:w86) -> (0:w83:errorcluster, 2:w78:dbl, 3:w84:refnum<file>)  [unwired: 3 in, 1 out]
          n83 = local write "Total USB resets"(w78) -> ()
          n84 = Close File(refnum=w84, error in=w83) -> (error out=w82:errorcluster)  [unwired: 1 out]
          n85 = local write "data file error"(w82) -> ()
        }
        frame #6 {
          # "get last saved jig cycles value from file"
          n86 = String To Path(string="c:\\crabtree\\Jig Cycles\\") -> (path=w100:path)
          n87 = Build Path(base path=w100, name or relative path="jigcycles.bin") -> (appended path=w98:path)
          n88 = Create Folder(path (use dialog)=w100) -> (error out=w102:errorcluster)  [unwired: 2 in, 2 out]
          n89 = call <vilib>:"Clear Errors.vi"("error in (no error)"=w102) -> ()  [unwired: 5 in, 2 out]
          n90 = Open/Create/Replace File(file path (use dialog)=w98) -> (refnum out=w96:refnum<file>, error out=w97:errorcluster)  [unwired: 5 in, 1 out]
          n91 = Read from Binary File(5:T8 {"LAB01-1"=0.0, "LAB01-2"=0.0, "LAB02-1"=0.0, "LAB02-2"=0.0, "LAB03-1"=0.0, "LAB03-2"=0.0, "LAB04-1"=0.0, "LAB04-2"=0.0, "LAB05-1"=0.0, "LAB05-2"=0.0} ("JIG RELAY CYCLES"), 8:w97, 11:w96) -> (0:w94:errorcluster, 2:w91:T8, 3:w95:refnum<file>)  [unwired: 3 in, 1 out]
          n92 = local write "JIG RELAY CYCLES"(w91) -> ()
          n93 = Close File(refnum=w95, error in=w94) -> (error out=w93:errorcluster)  [unwired: 1 out]
          n94 = local write "data file error"(w93) -> ()
        }
        frame #7 {
          # "get mail settings"
          n95 = local read "Auto Mail Send"() -> (w106:bool)
          n96 = local read "MAIL SETTINGS"() -> (w110:T7)
          n97 = String To Path(string="c:\\crabtree\\Set Up\\") -> (path=w118:path)
          n98 = Build Path(base path=w118, name or relative path="mail.bin") -> (appended path=w116:path)
          n99 = Create Folder(path (use dialog)=w118) -> (error out=w120:errorcluster)  [unwired: 2 in, 2 out]
          n100 = Bundle("MAIL SETTINGS"=w110, "Auto Mail Send"=w106, "") -> (w109:T23)  [unwired: 1 in]
          n101 = call <vilib>:"Clear Errors.vi"("error in (no error)"=w120) -> ()  [unwired: 5 in, 2 out]
          n102 = Open/Create/Replace File(file path (use dialog)=w116) -> (refnum out=w114:refnum<file>, error out=w115:errorcluster)  [unwired: 5 in, 1 out]
          n103 = Read from Binary File(5:w109, 8:w115, 11:w114) -> (0:w112:errorcluster, 2:w108:T23, 3:w113:refnum<file>)  [unwired: 3 in, 1 out]
          n104 = Unbundle(w108) -> ("MAIL SETTINGS"=w107:T7, "Auto Mail Send"=w105:bool, w104:string)
          n105 = local write "Auto Mail Send"(w105) -> ()
          n106 = local write "TO (string):"(w104) -> ()
          n107 = local write "MAIL SETTINGS"(w107) -> ()
          n108 = Close File(refnum=w113, error in=w112) -> (error out=w111:errorcluster)  [unwired: 1 out]
          n109 = local write "data file error"(w111) -> ()
        }
        frame #8 {
          # "set display status if blank"
          n110 = local read "DISP LAB03-2"() -> (w150:T4)
          n111 = local read "DISP LAB03-1"() -> (w157:T4)
          n112 = local read "DISP LAB02-2"() -> (w164:T4)
          n113 = local read "DISP LAB01-2"() -> (w177:T4)
          n114 = local read "DISP LAB01-1"() -> (w186:T4)
          n115 = local read "DISP LAB02-1"() -> (w171:T4)
          n116 = Unbundle(w150) -> ("STATUS"=w152:string)  [unwired: 2 out]
          n117 = Unbundle(w157) -> ("STATUS"=w159:string)  [unwired: 2 out]
          n118 = Unbundle(w164) -> ("STATUS"=w166:string)  [unwired: 2 out]
          n119 = Unbundle(w171) -> ("STATUS"=w173:string)  [unwired: 2 out]
          n120 = Unbundle(w177) -> ("STATUS"=w180:string)  [unwired: 2 out]
          n121 = Unbundle(w186) -> ("STATUS"=w187:string)  [unwired: 2 out]
          n122 = Equal?(x="", y=w152) -> (x = y?=w154:bool)
          n123 = Equal?(x="", y=w159) -> (x = y?=w161:bool)
          n124 = Equal?(x="", y=w166) -> (x = y?=w168:bool)
          n125 = Equal?(x="", y=w173) -> (x = y?=w175:bool)
          n126 = Equal?(x="", y=w180) -> (x = y?=w182:bool)
          n127 = Equal?(x="", y=w187) -> (x = y?=w189:bool)
          n128 = Select(t="STOP", s=w154, f=w152) -> (s? t:f=w151:string)
          n129 = Select(t="STOP", s=w161, f=w159) -> (s? t:f=w158:string)
          n130 = Select(t="STOP", s=w168, f=w166) -> (s? t:f=w165:string)
          n131 = Select(t="STOP", s=w175, f=w173) -> (s? t:f=w172:string)
          n132 = Select(t="STOP", s=w182, f=w180) -> (s? t:f=w179:string)
          n133 = Select(t="STOP", s=w189, f=w187) -> (s? t:f=w185:string)
          n134 = Bundle(cluster=w150, "STATUS"=w151) -> (w149:T4)  [unwired: 2 in]
          n135 = Bundle(cluster=w157, "STATUS"=w158) -> (w156:T4)  [unwired: 2 in]
          n136 = Bundle(cluster=w164, "STATUS"=w165) -> (w163:T4)  [unwired: 2 in]
          n137 = Bundle(cluster=w171, "STATUS"=w172) -> (w170:T4)  [unwired: 2 in]
          n138 = Bundle(cluster=w177, "STATUS"=w179) -> (w178:T4)  [unwired: 2 in]
          n139 = Bundle(cluster=w186, "STATUS"=w185) -> (w184:T4)  [unwired: 2 in]
          n140 = local write "DISP LAB01-2"(w178) -> ()
          n141 = local write "DISP LAB01-1"(w184) -> ()
          n142 = local write "DISP LAB02-1"(w170) -> ()
          n143 = local write "DISP LAB03-1"(w156) -> ()
          n144 = local write "DISP LAB02-2"(w163) -> ()
          n145 = local write "DISP LAB03-2"(w149) -> ()
          n146 = local read "DISP LAB05-2"() -> (w122:T4)
          n147 = local read "DISP LAB05-1"() -> (w129:T4)
          n148 = local read "DISP LAB04-2"() -> (w131:T4)
          n149 = local read "DISP LAB04-1"() -> (w133:T4)
          n150 = Unbundle(w122) -> ("STATUS"=w124:string)  [unwired: 2 out]
          n151 = Unbundle(w129) -> ("STATUS"=w135:string)  [unwired: 2 out]
          n152 = Unbundle(w131) -> ("STATUS"=w140:string)  [unwired: 2 out]
          n153 = Unbundle(w133) -> ("STATUS"=w145:string)  [unwired: 2 out]
          n154 = Equal?(x="", y=w124) -> (x = y?=w126:bool)
          n155 = Equal?(x="", y=w135) -> (x = y?=w137:bool)
          n156 = Equal?(x="", y=w140) -> (x = y?=w142:bool)
          n157 = Equal?(x="", y=w145) -> (x = y?=w147:bool)
          n158 = Select(t="STOP", s=w126, f=w124) -> (s? t:f=w123:string)
          n159 = Select(t="STOP", s=w137, f=w135) -> (s? t:f=w134:string)
          n160 = Select(t="STOP", s=w142, f=w140) -> (s? t:f=w139:string)
          n161 = Select(t="STOP", s=w147, f=w145) -> (s? t:f=w144:string)
          n162 = Bundle(cluster=w122, "STATUS"=w123) -> (w121:T4)  [unwired: 2 in]
          n163 = Bundle(cluster=w129, "STATUS"=w134) -> (w128:T4)  [unwired: 2 in]
          n164 = Bundle(cluster=w131, "STATUS"=w139) -> (w130:T4)  [unwired: 2 in]
          n165 = Bundle(cluster=w133, "STATUS"=w144) -> (w132:T4)  [unwired: 2 in]
          n166 = local write "DISP LAB05-2"(w121) -> ()
          n167 = local write "DISP LAB05-1"(w128) -> ()
          n168 = local write "DISP LAB04-1"(w132) -> ()
          n169 = local write "DISP LAB04-2"(w130) -> ()
        }
        frame #9 {
          w194 = 0
          w191 = FALSE
          # "initialise analog error control"
          n170 = local write "Resets Done"(0) -> ()
          n171 = local write "Auto Reset"(TRUE) -> ()
          n172 = local write "Er USB#0"(w194) -> ()
          n173 = local write "Er USB#1"(w194) -> ()
          n174 = local write "Er USB#2"(w194) -> ()
          n175 = local write "Analog error"(w191) -> ()
          n176 = local write "Reset Measuring"(w191) -> ()
          n177 = local write "Error USB #0"(w191) -> ()
          n178 = local write "Reset Error"(w191) -> ()
          n179 = local write "Error USB #1"(w191) -> ()
          n180 = local write "Error USB #2"(w191) -> ()
          n181 = local write "stop"(w191) -> ()
          n182 = local write "stop all"(w191) -> ()
        }
        frame #10 {
          # "get initial temperature values"
          n183 = stacked-sequence {
            frame #0 {
              w199 = T12 {"T1 Live"=20.0, "T1 Neut"=20.0, "T2 Live"=20.0, "T2 Neut"=20.0, "ID"=6.0, "ER"=10.0} ("LAB01 TEMP")
              n184 = local write "LAB deg C"(w199) -> ()
              n185 = global write "Global display 4.vi" "LAB deg C"(w199) -> ()
              n186 = local write "OFF amps"(1.5) -> ()
              n187 = local write "ON amps"(20.0) -> ()
              n188 = local write "VOLTS"(250.0) -> ()
              n189 = local write "PF"(0.5) -> ()
            }
            frame #1 {
              n190 = for {
                N: 3 -> [_]
                w245 = TRUE
                n191 = local read "Simulate"() -> (w207:bool)
                n192 = local write "Temp read loop"(0) -> ()
                n193 = case shown="True" w207 {
                  frame False {
                  }
                  frame True {
                    w247 = 20
                    n194 = local write "Ambient Volts"(2.92) -> ()
                    n195 = global write "Global display 3.vi" "Ref deg C"(w247) -> ()
                    n196 = local write "Ref deg C"(w247) -> ()
                  }
                }
